vi "Test Serializer.FlattenedString.vi"(8 "error in (no error)":errorcluster) -> (0 "error out":errorcluster)   [LabVIEW 2013]
uses:
  source/Serializer.FlattenedString/Serializer.FlattenedString.lvclass
  <vilib>/addons/_JKI Toolkits/Caraya/classes/Assert/Assert Equal Value and Type_Variant.vi
  <vilib>/addons/_JKI Toolkits/Caraya/classes/Assert/Assert Error.vi
  <vilib>/addons/_JKI Toolkits/Caraya/classes/Assert/Assert.lvclass
  source/Serializer/Serializer.lvclass
  <vilib>/addons/_JKI Toolkits/Caraya/classes/Test/Test.lvclass
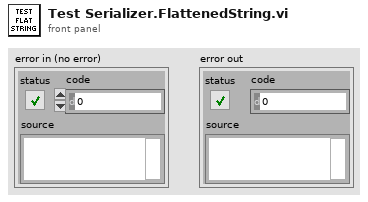
[diagram p1: front panel]
types:
  T1 = cluster{"error":errorcluster, "EnumU16":enum16{"A", "B", "C"}, "Value":dbl, "ArrayUnnamedElement":dbl[]}
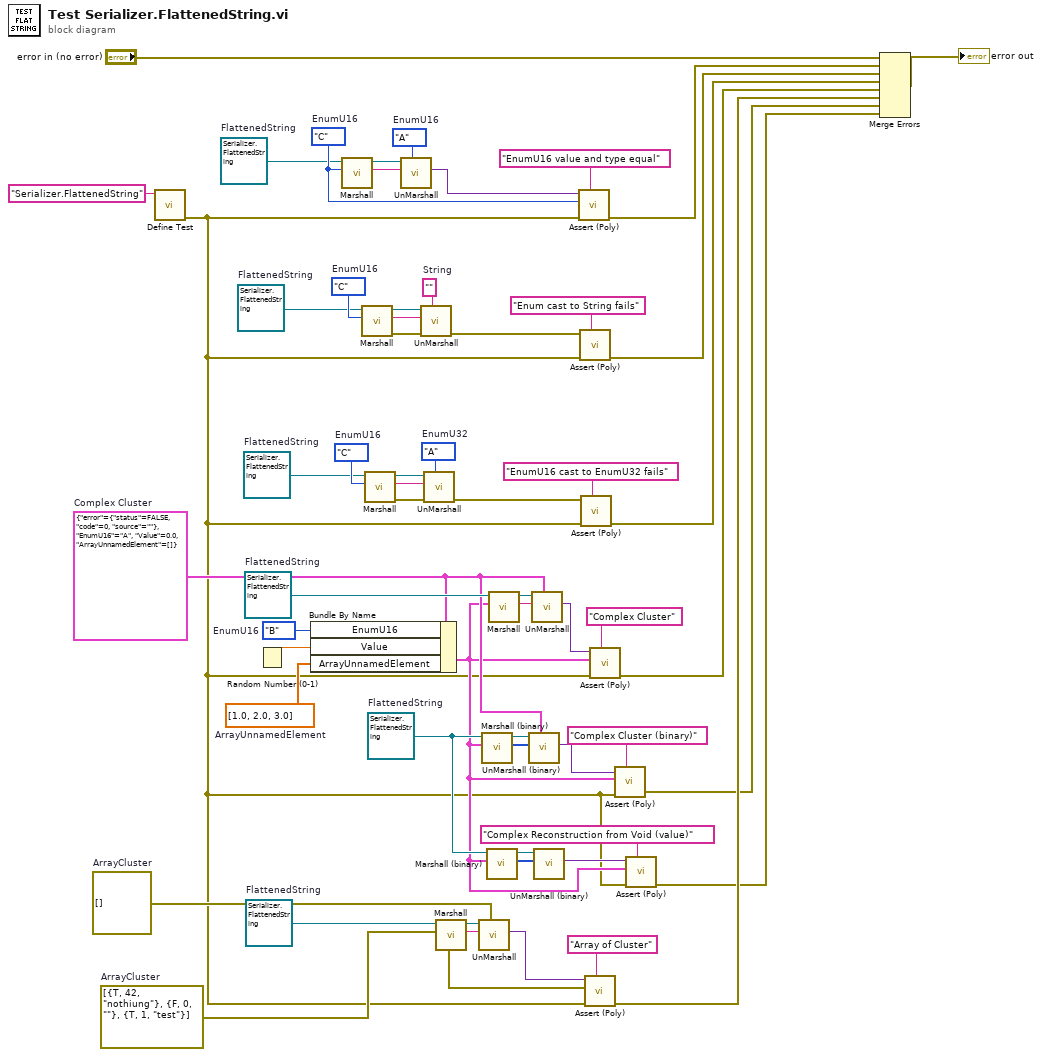
[diagram p0: block diagram]
diagram:
  w6 = refnum<class "Serializer.FlattenedString.lvclass"> refnum  # FlattenedString
  w15 = refnum<class "Serializer.FlattenedString.lvclass"> refnum  # FlattenedString
  w16 = refnum<class "Serializer.FlattenedString.lvclass"> refnum  # FlattenedString
  w17 = refnum<class "Serializer.FlattenedString.lvclass"> refnum  # FlattenedString
  w18 = refnum<class "Serializer.FlattenedString.lvclass"> refnum  # FlattenedString
  w19 = refnum<class "Serializer.FlattenedString.lvclass"> refnum  # FlattenedString
  w21 = errorcluster[] [{"status"=TRUE, "code"=42, "source"="nothiung"}, {"status"=FALSE, "code"=0, "source"=""}, {"status"=TRUE, "code"=1, "source"="test"}]  # ArrayCluster
  w22 = errorcluster[] []  # ArrayCluster
  w27 = dbl[] [1.0, 2.0, 3.0]  # ArrayUnnamedElement
  w29 = enum16{"A", "B", "C"}."B"  # EnumU16
  w12 = T1 {"error"={"status"=FALSE, "code"=0, "source"=""}, "EnumU16"=enum."A", "Value"=0.0, "ArrayUnnamedElement"=[]}  # Complex Cluster
  w35 = enum32{"A", "B", "C"}."A"  # EnumU32
  w40 = enum16{"A", "B", "C"}."C"  # EnumU16
  w48 = ""  # String
  w46 = enum16{"A", "B", "C"}."C"  # EnumU16
  w57 = enum16{"A", "B", "C"}."A"  # EnumU16
  w59 = enum16{"A", "B", "C"}."C"  # EnumU16
  n1 = call <vilib>:"Define Test.vi"("Label (VI Title)"="Serializer.FlattenedString") -> ("error out"=w3:errorcluster)  [unwired: 10 in]
  n2 = Random Number (0-1)() -> (number: 0 to 1=w28:dbl)
  n3 = Bundle By Name(cluster=w12, "EnumU16"=w29, "Value"=w28, "ArrayUnnamedElement"=w27) -> (w4:T1)
  n4 = call "Marshall.vi"("Variant"=w59, "Serializer in"=w19) -> ("String"=w56:string, "Serializer out"=w55:refnum<class "Serializer.FlattenedString.lvclass">)  [unwired: 7 in, 1 out]
  n5 = call "Marshall.vi"("Variant"=w46, "Serializer in"=w18) -> ("error out"=w43:errorcluster, "String"=w49:string, "Serializer out"=w50:refnum<class "Serializer.FlattenedString.lvclass">)  [unwired: 7 in]
  n6 = call "Marshall.vi"("Variant"=w40, "Serializer in"=w17) -> ("error out"=w42:errorcluster, "String"=w38:string, "Serializer out"=w37:refnum<class "Serializer.FlattenedString.lvclass">)  [unwired: 7 in]
  n7 = call "UnMarshall.vi"("Type"=w57, "String"=w56, "Serializer in"=w55) -> ("Variant"=w58:variant)  [unwired: 6 in, 2 out]
  n8 = call "UnMarshall.vi"("Type"=w48, "error in (no error)"=w43, "String"=w49, "Serializer in"=w50) -> ("error out"=w44:errorcluster)  [unwired: 5 in, 2 out]
  n9 = call "UnMarshall.vi"("Type"=w35, "error in (no error)"=w42, "String"=w38, "Serializer in"=w37) -> ("error out"=w41:errorcluster)  [unwired: 5 in, 2 out]
  n10 = call "Marshall.vi"("Variant"=w21, "Serializer in"=w15) -> ("String"=w24:string, "Serializer out"=w23:refnum<class "Serializer.FlattenedString.lvclass">)  [unwired: 7 in, 1 out]
  n11 = call "UnMarshall.vi"("Type"=w22, "String"=w24, "Serializer in"=w23) -> ("Variant"=w25:variant)  [unwired: 6 in, 2 out]
  n12 = call "Marshall (binary).vi"("Variant"=w4, "Serializer in"=w6) -> ("Bytes"=w14:u8[], "Serializer out"=w13:refnum<class "Serializer.FlattenedString.lvclass">)  [unwired: 7 in, 1 out]
  n13 = call "Marshall (binary).vi"("Variant"=w4, "Serializer in"=w6) -> ("Bytes"=w7:u8[], "Serializer out"=w8:refnum<class "Serializer.FlattenedString.lvclass">)  [unwired: 7 in, 1 out]
  n14 = call "Marshall.vi"("Variant"=w4, "Serializer in"=w16) -> ("String"=w33:string, "Serializer out"=w34:refnum<class "Serializer.FlattenedString.lvclass">)  [unwired: 7 in, 1 out]
  n15 = call "UnMarshall (binary).vi"("Type"=w12, "Bytes"=w14, "Serializer in"=w13) -> ("Variant"=w9:variant)  [unwired: 6 in, 2 out]
  n16 = call "UnMarshall.vi"("Type"=w12, "String"=w33, "Serializer in"=w34) -> ("Variant"=w32:variant)  [unwired: 6 in, 2 out]
  n17 = call "UnMarshall (binary).vi"("Bytes"=w7, "Serializer in"=w8) -> ("Variant"=w5:variant)  [unwired: 7 in, 2 out]
  n18 = call-poly <vilib>:"Assert (Poly).vi"("Label"="EnumU16 value and type equal", "error in (no error)"=w3, "Y"=w59, "X"=w58) -> ("error out"=w51:errorcluster)  [unwired: 7 in]
  n19 = call-poly <vilib>:"Assert (Poly).vi"("Label"="Enum cast to String fails", "error in (no error)"=w3, "Error?"=w44) -> ("error out"=w45:errorcluster)  [unwired: 8 in]
  n20 = call-poly <vilib>:"Assert (Poly).vi"("Label"="EnumU16 cast to EnumU32 fails", "error in (no error)"=w3, "Error?"=w41) -> ("error out"=w36:errorcluster)  [unwired: 8 in]
  n21 = call-poly <vilib>:"Assert (Poly).vi"("Label"="Array of Cluster", "error in (no error)"=w3, "Y"=w21, "X"=w25) -> ("error out"=w20:errorcluster)  [unwired: 7 in]
  n22 = call-poly <vilib>:"Assert (Poly).vi"("Label"="Complex Cluster", "error in (no error)"=w3, "Y"=w4, "X"=w32) -> ("error out"=w30:errorcluster)  [unwired: 7 in]
  n23 = call-poly <vilib>:"Assert (Poly).vi"("Label"="Complex Cluster (binary)", "error in (no error)"=w3, "Y"=w4, "X"=w9) -> ("error out"=w10:errorcluster)  [unwired: 7 in]
  n24 = call-poly <vilib>:"Assert (Poly).vi"("Label"="Complex Reconstruction from Void (value)", "error in (no error)"=w3, "Y"=w4, "X"=w5) -> ("error out"=w2:errorcluster)  [unwired: 7 in]
  n25 = Merge Errors("error in (no error)", w51, w45, w36, w30, w20, w10, w2) -> (→"error out":errorcluster)
